vi "Product Cluster to String Array.vi"(11 "Products Cluster Array":T1[](array[typedef])) -> (3 "Products String Array":string[][](array[string]))   [LabVIEW 2020, in "Product Selecting Pane.lvlib"]
doc: "Converts a Product Cluster Array into a 2D string array to be displayed in a list on the UI."
uses:
  Product Selecting Pane.lvlib
  SQLITE Inventory/Invetory Data Type.ctl
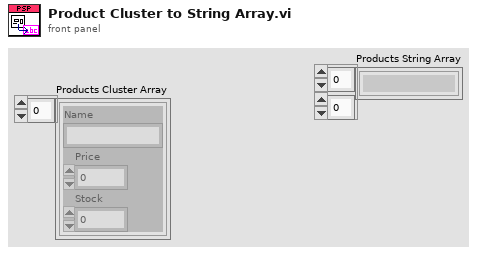
[diagram p1: front panel]
types:
  T1 = typedef "Invetory Data Type.ctl" = cluster{"Name":string, "Price":dbl, "Stock":dbl}
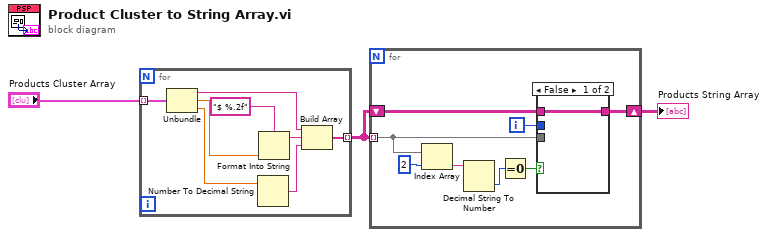
[diagram p0: block diagram]
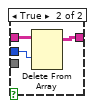
[diagram p2: hidden frame]
diagram:
  n1 = for {
    tunnel: "Products Cluster Array" -> [w11] mode=indexing
    tunnel: [w4] -> w2 mode=indexing
    n2 = Unbundle(w11) -> ("Name"=w7:string, "Price"=w10:dbl, "Stock"=w8:dbl)
    n3 = Number To Decimal String(number=w8) -> (decimal integer string=w5:string)  [unwired: 1 in]
    n4 = Format Into String(format string="$ %.2f", w10) -> (resulting string=w6:string)  [unwired: 2 in, 1 out]
    n5 = Build Array(w7, w6, w5) -> (w4:string[])
  }
  n6 = for {
    tunnel: w2 -> [w16] mode=indexing
    shift-right: [w15] -> w1
    shift-left: w2 -> [w14]
    i -> [w13]
    n7 = Index Array(array=w16, index=2) -> (element=w18:string)
    n8 = Decimal String To Number(string=w18) -> (number=w12:i32)  [unwired: 2 in, 1 out]
    n9 = Equal To 0?(x=w12) -> (x = 0?=w17:bool)
    n10 = case shown="False" w17 {
      tunnel: w16 -> [_ _]
      tunnel: [w20 w21] -> w15
      tunnel: w14 -> [w20 w23]
      tunnel: w13 -> [_ w22]
      frame False {
      }
      frame True {
        n11 = Delete From Array(array=w23, index (row)=w22) -> (array with subset deleted=w21:string[][])  [unwired: 2 in, 1 out]
      }
    }
  }
  "Products String Array" <- w1
